vi "Error Query.vi"(0 "VISA resource name":refnum<visa-resource-name>, 11 "error in (no error)":errorcluster {"code" format="%.0x"}) -> (4 "VISA resource name out":refnum<visa-resource-name>, 8 "Error":i32, 10 "Error Message":string, 15 "error out":errorcluster {"code" format="%.0x"})   [LabVIEW 2018, in "Agilent N6700 Series.lvlib"]
doc: "Reads an error code and a message from the instrument's error queue.\n\n<b>Note:</b>\nThis VI is called automatically by most driver VIs so it is not usually necessary to call this in an application."
uses:
  Agilent N6700 Series.lvlib
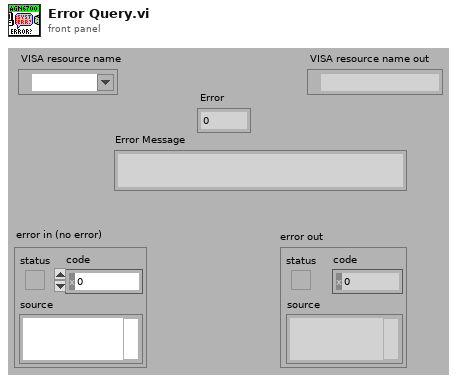
[diagram p1: front panel]
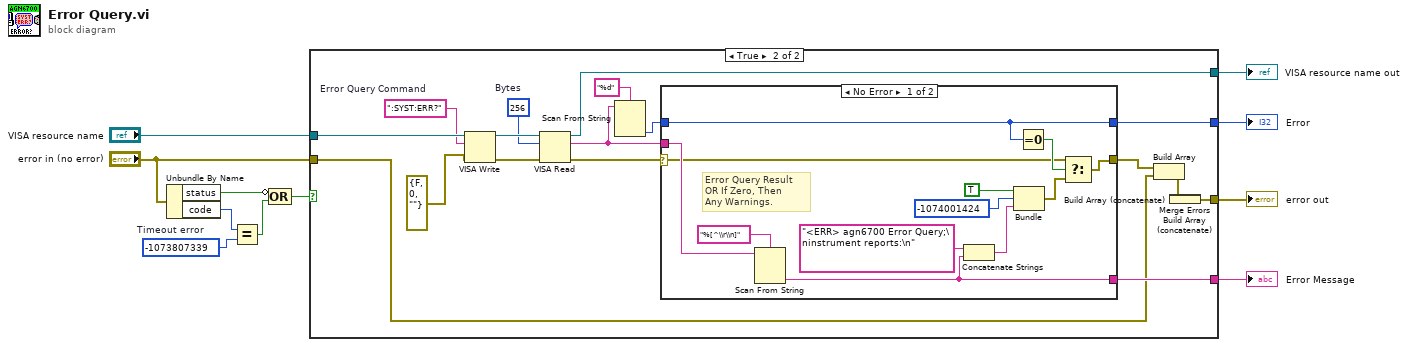
[diagram p0: block diagram]
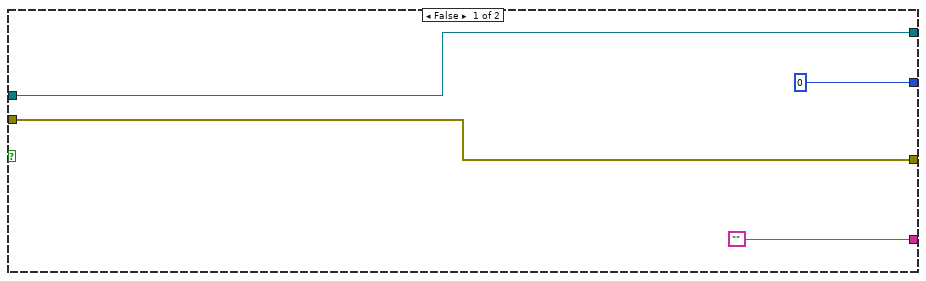
[diagram p2: hidden frame]
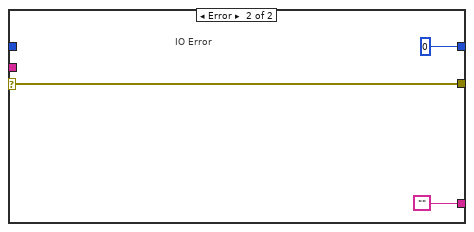
[diagram p3: hidden frame]
diagram:
  w4 = -1073807339  # Timeout error
  n1 = Unbundle By Name("error in (no error)") -> ("status"=w5:bool, "code"=w2:i32)
  n2 = Equal?(x=w2, y=w4) -> (x = y?=w3:bool)
  n3 = Compound Arithmetic op=OR(invert w5, w3) -> (w1:bool)
  n4 = case shown="True" w1 {
    tunnel: ["" ("Empty String Constant") w34] -> w11
    tunnel: [0 w33] -> w10
    tunnel: [w15 w32] -> w9
    tunnel: "VISA resource name" -> [w15 w31]
    tunnel: "error in (no error)" -> [w12 w24]
    tunnel: [w12 w23] -> w7
    frame False {
    }
    frame True {
      w29 = u32 256  # Bytes
      w27 = ":SYST:ERR?"  # Error Query Command
      n5 = VISA Write(VISA resource name=w31, write buffer=w27, error in (no error)=errorcluster {"status"=FALSE, "code"=0, "source"=""}) -> (VISA resource name out=w30:refnum<visa-resource-name>, error out=w28:errorcluster)  [unwired: 1 out]
      n6 = VISA Read(VISA resource name=w30, byte count=w29, error in (no error)=w28) -> (VISA resource name out=w32:refnum<visa-resource-name>, read buffer=w22:string, error out=w19:errorcluster)  [unwired: 1 out]
      n7 = Scan From String(format string="%d", input string=w22) -> (output 1=w20:i32)  [unwired: 3 in, 3 out]
      n8 = case shown="No Error" w19 {
        selector: w19 -> [w35 w47]
        tunnel: w22 -> [w37 _]
        tunnel: [w42 w47] -> w25
        tunnel: [w38 "" ("Empty String Constant")] -> w34
        tunnel: [w36 0] -> w33
        tunnel: w20 -> [w36 _]
        frame No Error {
          # "Error Query Result\nOR If Zero, Then\nAny Warnings."
          n9 = Scan From String(format string="%[^\\r\\n]", input string=w37) -> (output 1=w38:string)  [unwired: 3 in, 3 out]
          n10 = Concatenate Strings("<ERR> agn6700 Error Query;\ninstrument reports:\n" ("Source"), w38) -> (w44:string)
          n11 = Bundle("Status"=TRUE, "Code"=-1074001424, w44) -> (w43:cluster{"Status":bool, "Code":i32, string})  [unwired: 1 in]
          n12 = Equal To 0?(x=w36) -> (x = 0?=w40:bool)
          n13 = Select(t=w35, s=w40, f=w43) -> (s? t:f=w42:errorcluster)
        }
        frame Error {
          # "IO Error"
        }
      }
      n14 = Build Array(w25, w24) -> (w18:errorcluster[])
      n15 = Build Array (concatenate)(w18) -> (w17:errorcluster[])
      n16 = Build Array (concatenate)(w17) -> (w16:errorcluster[])
      n17 = Merge Errors(w16) -> (w23:errorcluster)
    }
  }
  "Error Message" <- w11
  "Error" <- w10
  "VISA resource name out" <- w9
  "error out" <- w7
